vi "bypass.vi"(5 "Run VI":bool, 6 "Set # of Turns Open":dbl, 8 "stop":bool, 10 "position":refnum<vi>) -> ()   [LabVIEW 2015]
uses:
  <vilib>/Utility/config.llb/Read Key (String).vi
  <vilib>/Utility/config.llb/Read Key (Path).vi
  subvi_motor/global_motor.vi
  <vilib>/Utility/config.llb/NI_LVConfig.lvlib
panel:
  in  "Motor Enabled":bool=TRUE
  in  "Recalibrate":bool
  in  "Current Position":dbl
  out "Motor Connected":bool
  in  "Enable Advanced Controls":bool
  in  "Log Data?":bool
  out "Valve Position":dynamicdata(graph)
  out "# of Turns Open":dbl
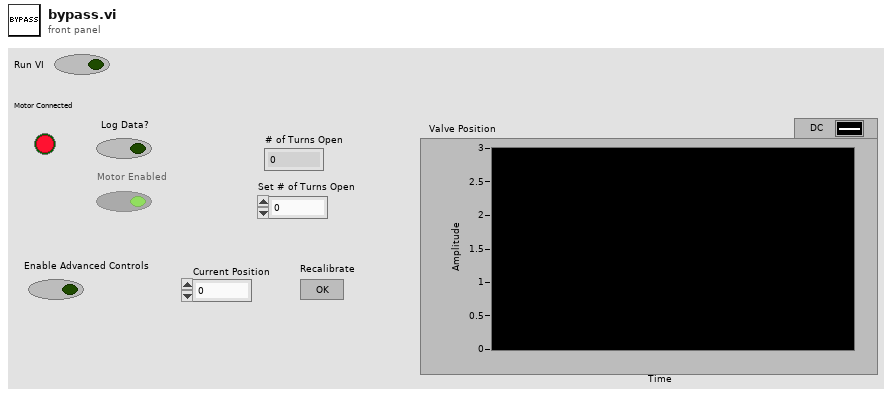
[diagram p1: front panel]
types:
  T1 = enum16{"open", "replace", "create", "open or create", "replace or create", "replace or create with confirmation"}
  T2 = enum8{"Enabled", "Disabled", "Disabled and Grayed Out"}
  T3 = typedef "NI_LVConfig.lvlib/Config Data RefNum.ctl" = refnum<k1>
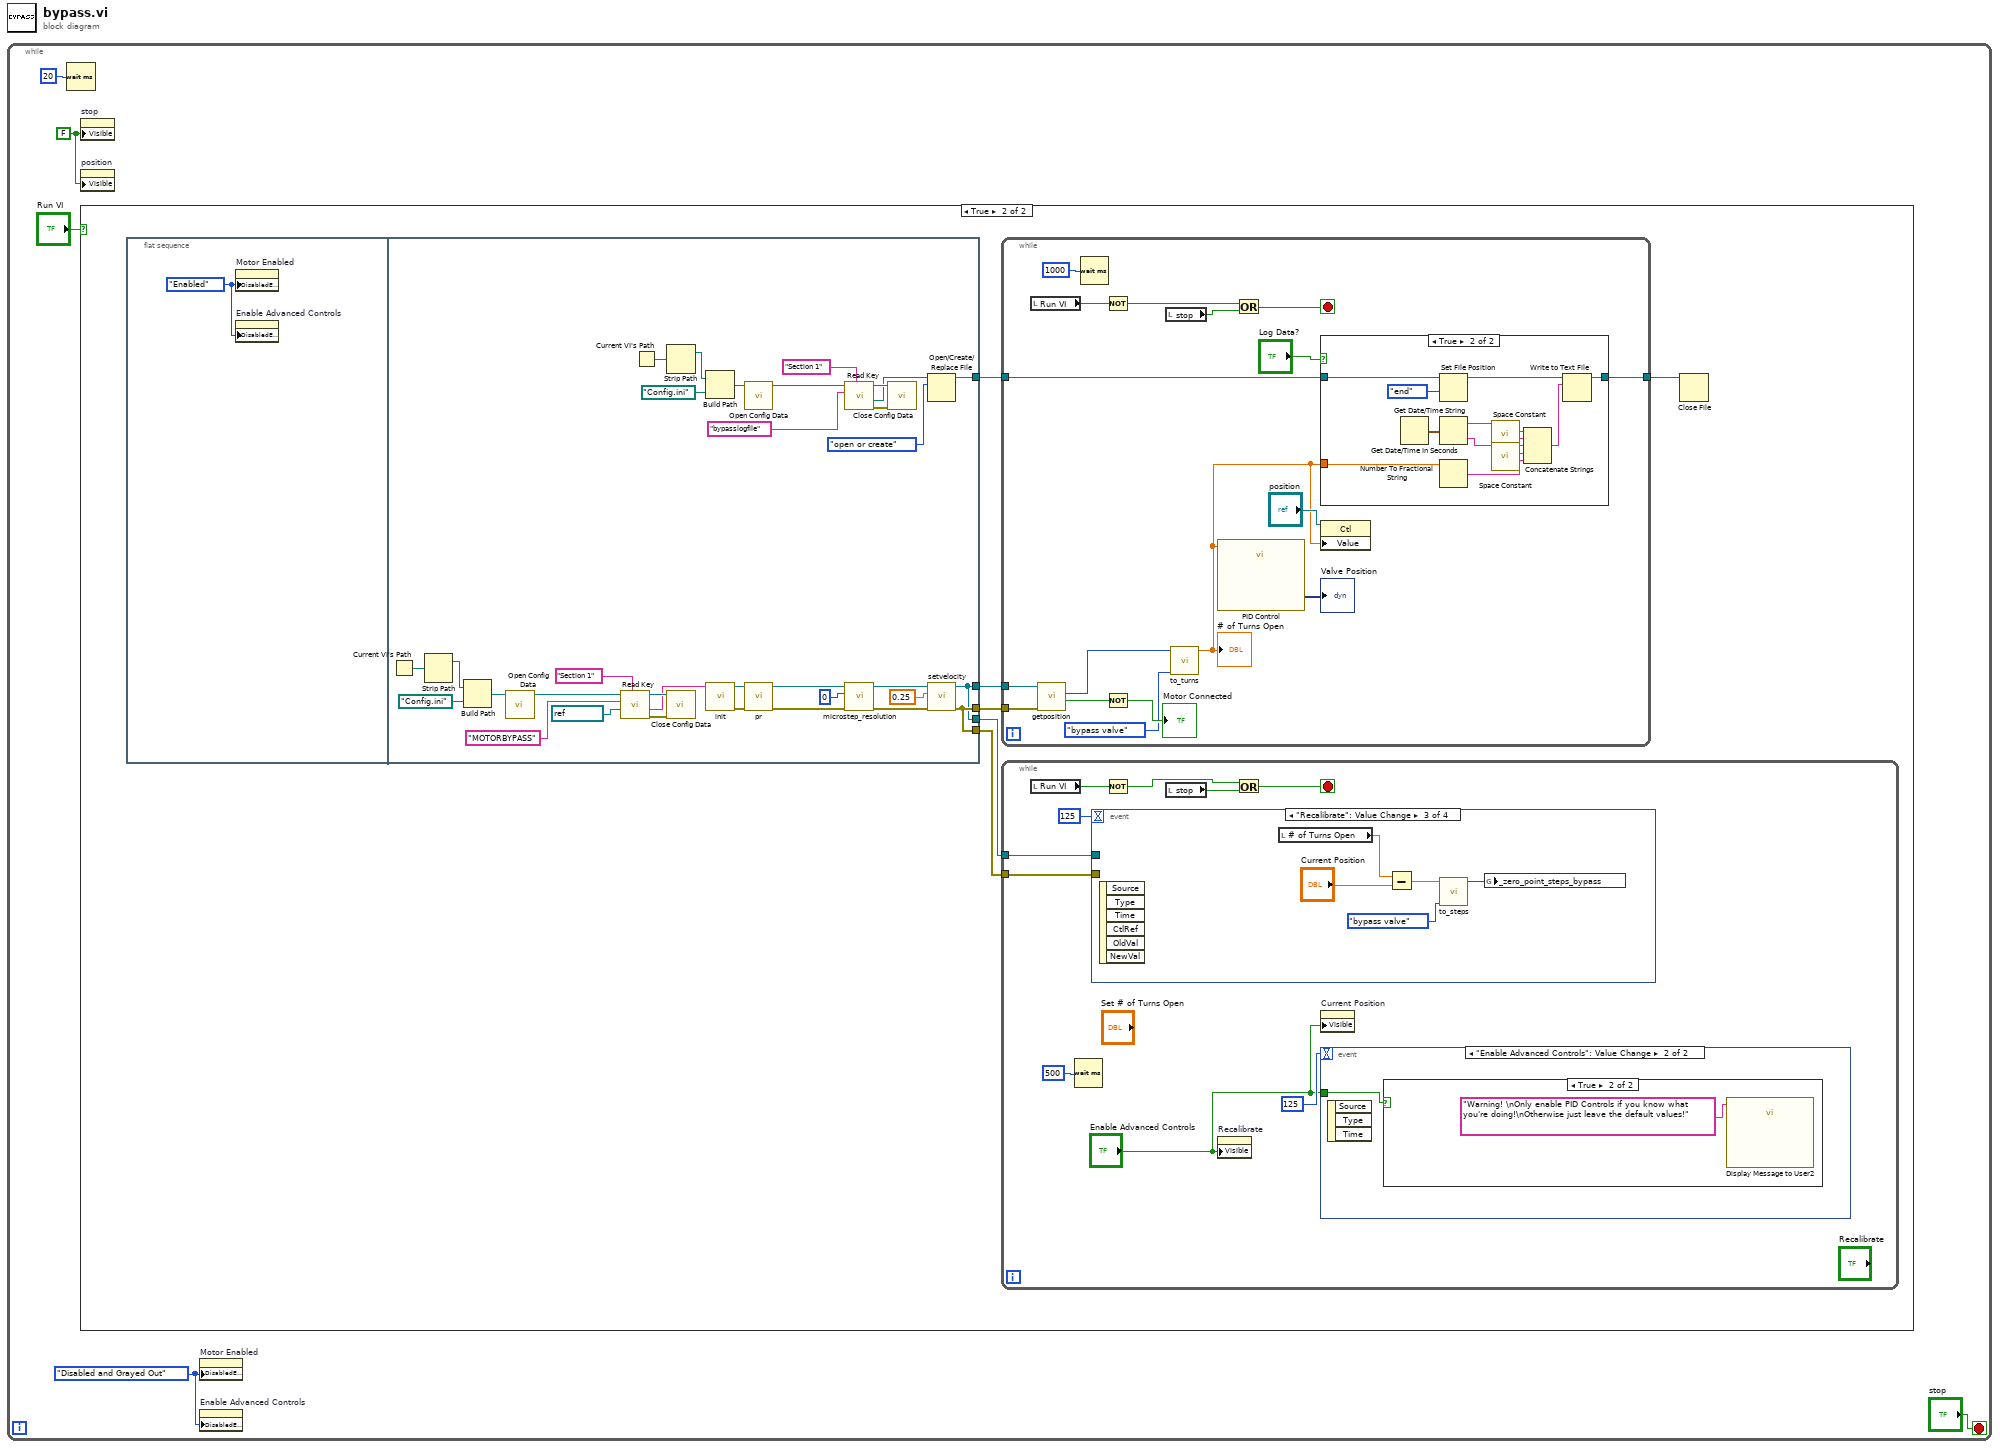
[diagram p0: block diagram]
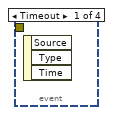
[diagram p4: hidden frame]
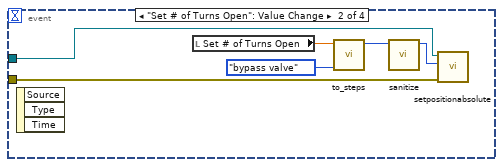
[diagram p5: hidden frame]
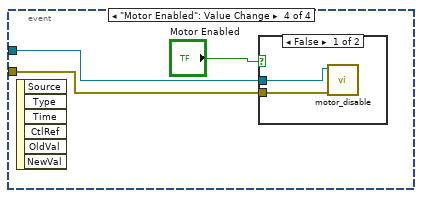
[diagram p6: hidden frame]
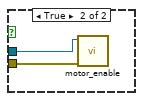
[diagram p7: hidden frame]
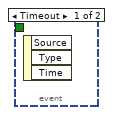
[diagram p8: hidden frame]
diagram:
  n1 = while {
    stop <- "stop" stop-if-true
    w1 = FALSE ("Visible")
    w2 = T2."Disabled and Grayed Out" ("Disabled")
    n2 = Wait (ms)(milliseconds to wait=u32 20) -> ()  [unwired: 1 out]
    n3 = property on="stop" class="Bool (strict)"("Visible"=w1) -> ()  [unwired: 2 in, 2 out]
    n4 = property on="position" class="LVObjRef (strict)"("Visible"=w1) -> ()  [unwired: 2 in, 2 out]
    n5 = case shown="True" "Run VI" {
      frame False {
      }
      frame True {
        n6 = flat-sequence {
          tunnel: [w44] -> w11
          tunnel: [w44] -> w10
          tunnel: [w43] -> w9
          tunnel: [w43] -> w8
          tunnel: [w39] -> w7
          frame #0 {
            w12 = T2."Enabled" ("Disabled")
            n7 = property on="Motor Enabled" class="Bool (strict)"("DisabledEnum"=w12) -> ()  [unwired: 2 in, 2 out]
            n8 = property on="Enable Advanced Controls" class="Bool (strict)"("DisabledEnum"=w12) -> ()  [unwired: 2 in, 2 out]
          }
          frame #1 {
            n9 = Current VI's Path() -> (path=w25:path)
            n10 = Strip Path(path=w25) -> (stripped path=w24:path)  [unwired: 1 out]
            n11 = Build Path(base path=w24, name or relative path=path "Config.ini" ("default name")) -> (appended path=w28:path)
            n12 = call <vilib>:"Open Config Data.vi"("configuration file path"=w28) -> ("refnum"=w33:T3)  [unwired: 8 in, 2 out]
            n13 = call-poly <vilib>:"Read Key.vi"("section"="Section 1", "default value"=refnum<visa-resource-name> "COM5" ("VISA resource name"), "key"="MOTORBYPASS", "refnum"=w33) -> ("error out"=w27:errorcluster, "value"=w23:string, "refnum out"=w31:T3)  [unwired: 4 in, 1 out]
            n14 = Current VI's Path() -> (path=w15:path)
            n15 = Strip Path(path=w15) -> (stripped path=w14:path)  [unwired: 1 out]
            n16 = call <vilib>:"Close Config Data.vi"("error in (no error)"=w27, "refnum"=w31) -> ()  [unwired: 8 in, 2 out]
            n17 = Build Path(base path=w14, name or relative path=path "Config.ini" ("default name")) -> (appended path=w17:path)
            n18 = call "init.vi"("VISA resource name"=w23) -> ("error out"=w35:errorcluster, "VISA resource name 2"=w37:refnum<visa-resource-name>)  [unwired: 9 in]
            n19 = call <vilib>:"Open Config Data.vi"("configuration file path"=w17) -> ("refnum"=w22:T3)  [unwired: 8 in, 2 out]
            n20 = call "pr.vi"("error in (no error)"=w35, "VISA resource name"=w37) -> ("error out"=w34:errorcluster, "VISA resource name 2"=w36:refnum<visa-resource-name>)  [unwired: 8 in]
            n21 = call-poly <vilib>:"Read Key.vi"("section"="Section 1", "key"="bypasslogfile", "refnum"=w22) -> ("error out"=w16:errorcluster, "value"=w13:path, "refnum out"=w20:T3)  [unwired: 5 in, 1 out]
            n22 = call "microstep_resolution.vi"("error in (no error)"=w34, "number"=0, "VISA in"=w36) -> ("error out"=w41:errorcluster, "VISA out"=w40:refnum<visa-resource-name>)  [unwired: 7 in]
            n23 = call <vilib>:"Close Config Data.vi"("error in (no error)"=w16, "refnum"=w20) -> ()  [unwired: 8 in, 2 out]
            n24 = Open/Create/Replace File(file path (use dialog)=w13, operation (0:open)=T1."open or create") -> (refnum out=w39:refnum<file>)  [unwired: 4 in, 2 out]
            n25 = call "setvelocity.vi"("error in (no error)"=w41, "Velocity"=0.25, "VISA in"=w40) -> ("error out"=w44:errorcluster, "VISA out"=w43:refnum<visa-resource-name>)  [unwired: 7 in]
          }
        }
        n26 = while {
          tunnel: w10 -> [w61]
          tunnel: w8 -> [w60]
          tunnel: w7 -> [w48]
          tunnel: [w47] -> w6
          stop <- w50 stop-if-true
          n27 = local read "Run VI"() -> (w54:bool)
          n28 = call "getposition.vi"("error in (no error)"=w61, "VISA resource name"=w60) -> ("Is Null?"=w57:bool, "Position"=w55:i32)  [unwired: 6 in, 2 out]
          n29 = Wait (ms)(milliseconds to wait=u32 1000) -> ()  [unwired: 1 out]
          n30 = Not(x=w54) -> (.not. x?=w51:bool)
          n31 = Not(x=w57) -> (.not. x?=→"Motor Connected":bool)
          n32 = local read "stop"() -> (w49:bool)
          n33 = call "to_turns.vi"("Radio Buttons"=enum32{"run valve", "bypass valve"}."bypass valve", "Steps"=w55) -> ("Turns"=w52:dbl)  [unwired: 9 in]
          "# of Turns Open" <- w52
          n34 = call "PID Control"("Offset"=w52) -> ("DC"=→"Valve Position":dynamicdata)  [unwired: 13 in, 1 out]
          n35 = Or(x=w51, y=w49) -> (x .or. y?=w50:bool)
          n36 = case shown="True" "Log Data?" {
            tunnel: w52 -> [_ w75]
            tunnel: w48 -> [w63 w70]
            tunnel: [w63 w69] -> w47
            frame False {
            }
            frame True {
              n37 = Get Date/Time In Seconds() -> (seconds since 1Jan1904=w68:timestamp)
              n38 = Set File Position(refnum=w70, from (0:start)=enum16{"start", "end", "current"}."end") -> (refnum out=w71:refnum<file>)  [unwired: 2 in, 1 out]
              n39 = Get Date/Time String(seconds (now)=w68) -> (date string=w66:string, time string=w67:string)  [unwired: 2 in]
              n40 = Number To Fractional String(number=w75) -> (F-format string=w64:string)  [unwired: 3 in]
              n41 = call <vilib>:"Space Constant.vi"() -> ("String"=w65:string)
              n42 = call <vilib>:"Space Constant.vi"() -> ("String"=w73:string)
              n43 = Concatenate Strings(w66, w65, w67, w73, w64) -> (w74:string)
              n44 = Write to Text File(file (use dialog)=w71, text=w74) -> (refnum out=w69:refnum<file>)  [unwired: 2 in, 2 out]
            }
          }
          n45 = property class="Ctl"(reference="position", "Value"=w52) -> ()  [unwired: 1 in, 2 out]
        }
        n46 = while {
          tunnel: w11 -> [w77]
          tunnel: w9 -> [w78]
          stop <- w81 stop-if-true
          n47 = local read "Run VI"() -> (w83:bool)
          n48 = Wait (ms)(milliseconds to wait=u32 500) -> ()  [unwired: 1 out]
          n49 = event shown="[2] \"Recalibrate\": Value Change" {
            selector: _ -> [_ _ _ _]
            dyn-events: _ -> [_ _ _ _]
            timeout: 125 -> [_ _ _ _]
            tunnel: w78 -> [_ w90 _ w99]
            tunnel: w77 -> [_ w89 _ w98]
            event Timeout {
              n50 = event-data() -> ()  [unwired: 1 in, 3 out]
            }
            event "Set # of Turns Open": Value Change {
              n51 = event-data() -> ()  [unwired: 1 in, 3 out]
              n52 = local read "Set # of Turns Open"() -> (w88:dbl)
              n53 = call "to_steps.vi"("Radio Buttons"=enum32{"run valve", "bypass valve"}."bypass valve", "Turns"=w88) -> ("Steps"=w87:i32)  [unwired: 9 in]
              n54 = call "sanitize.vi"("Input"=w87) -> ("Sanitized Input"=w91:i32)  [unwired: 10 in]
              n55 = call "setpositionabsolute.vi"("error in (no error)"=w89, "Position Aboslute"=w91, "VISA in"=w90) -> ()  [unwired: 7 in, 2 out]
            }
            event "Recalibrate": Value Change {
              n56 = event-data() -> ()  [unwired: 1 in, 6 out]
              n57 = local read "# of Turns Open"() -> (w94:dbl)
              n58 = Subtract(x=w94, y="Current Position") -> (x-y=w95:dbl)
              n59 = call "to_steps.vi"("Radio Buttons"=enum32{"run valve", "bypass valve"}."bypass valve", "Turns"=w95) -> ("Steps"=w96:i32)  [unwired: 9 in]
              n60 = global write "global_motor.vi" "_zero_point_steps_bypass"(w96) -> ()
            }
            event "Motor Enabled": Value Change {
              n61 = event-data() -> ()  [unwired: 1 in, 6 out]
              n62 = case shown="False" "Motor Enabled" {
                tunnel: w99 -> [w100 w103]
                tunnel: w98 -> [w101 w102]
                frame False {
                  n63 = call "motor_disable.vi"("error in (no error)"=w101, "VISA resource name"=w100) -> ()  [unwired: 8 in, 2 out]
                }
                frame True {
                  n64 = call "motor_enable.vi"("error in (no error)"=w102, "VISA resource name"=w103) -> ()  [unwired: 8 in, 2 out]
                }
              }
            }
          }
          n65 = Not(x=w83) -> (.not. x?=w82:bool)
          n66 = local read "stop"() -> (w80:bool)
          n67 = property on="Recalibrate" class="Bool"("Visible"="Enable Advanced Controls") -> ()  [unwired: 2 in, 2 out]
          n68 = Or(x=w82, y=w80) -> (x .or. y?=w81:bool)
          n69 = property on="Current Position" class="DigNum (strict)"("Visible"="Enable Advanced Controls") -> ()  [unwired: 2 in, 2 out]
          n70 = event shown="[1] \"Enable Advanced Controls\": Value Change" {
            selector: _ -> [_ _]
            dyn-events: _ -> [_ _]
            timeout: 125 -> [_ _]
            tunnel: "Enable Advanced Controls" -> [_ w104]
            event Timeout {
              n71 = event-data() -> ()  [unwired: 1 in, 3 out]
            }
            event "Enable Advanced Controls": Value Change {
              n72 = event-data() -> ()  [unwired: 1 in, 3 out]
              n73 = case shown="True" w104 {
                frame False {
                }
                frame True {
                  n74 = call "Display Message to User2"("Message"="Warning! \nOnly enable PID Controls if you know what you're doing!\nOtherwise just leave the default values!") -> ()  [unwired: 9 in, 2 out]
                }
              }
            }
          }
        }
        n75 = Close File(refnum=w6) -> ()  [unwired: 1 in, 2 out]
      }
    }
    n76 = property on="Motor Enabled" class="Bool (strict)"("DisabledEnum"=w2) -> ()  [unwired: 2 in, 2 out]
    n77 = property on="Enable Advanced Controls" class="Bool (strict)"("DisabledEnum"=w2) -> ()  [unwired: 2 in, 2 out]
  }
